vi "GPIB Bus Scan (for CCD).vi"(1 "Bus Timeout (mS)":i32=100) -> (0 "?":string)   [LabVIEW 2025]
doc: "Scans all primary addresses on the GPIB bus and reports status of devices found there.\nScott Hannahs, F. Bitter National Magnet Lab, April 1993\nAuthor: Scott Hannahs <sth@magnet.fsu.edu>\n\nThis software is licensed for use under the “MIT License\"\nCopyright (c) 2025 Scott Hannahs, sth@sth@magnet.sthnet.net\n\nPermission is hereby granted, free of charge, to any person obtaining a copy of this software and associated documentation files (the \"Software\"), to deal in the Software without restriction, including without limitation the rights to use, copy, modify, merge, publish, distribute, sublicense, and/or sell copies of the Software, and to permit persons to whom the Software is furnished to do so, subject to the following conditions: The above copyright notice and this permission notice shall be included in all copies or substantial portions of the Software.\n\nTHE SOFTWARE IS PROVIDED \"AS IS\", WITHOUT WARRANTY OF ANY KIND, EXPRESS OR IMPLIED, INCLUDING BUT NOT LIMITED TO THE WARRANTIES OF MERCHANTABILITY, FITNESS FOR A PARTICULAR PURPOSE AND NONINFRINGEMENT. IN NO EVENT SHALL THE AUTHORS OR COPYRIGHT HOLDERS BE LIABLE FOR ANY CLAIM, DAMAGES OR OTHER LIABILITY, WHETHER IN AN ACTION OF CONTRACT, TORT OR OTHERWISE, ARISING FROM, OUT OF OR IN CONNECTION WITH THE SOFTWARE OR THE USE OR OTHER DEALINGS IN THE SOFTWARE."
panel:
  in  "stop":bool
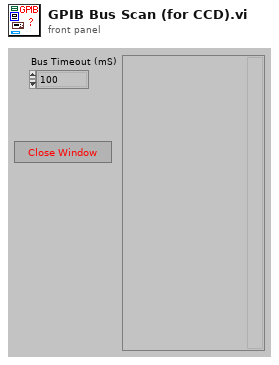
[diagram p1: front panel]
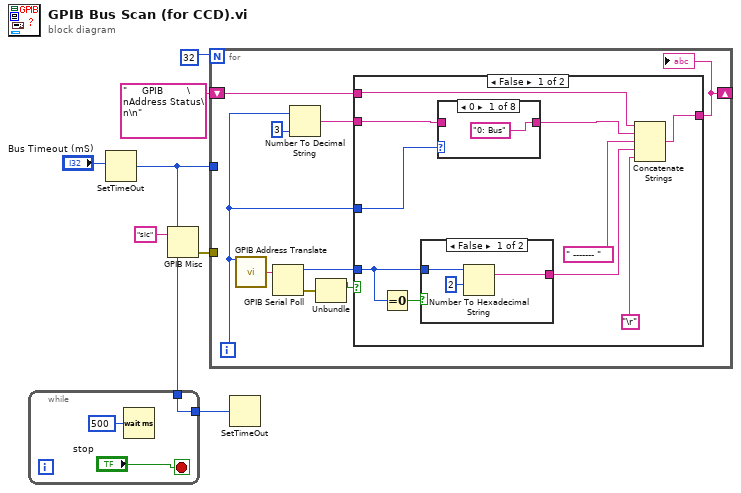
[diagram p0: block diagram]
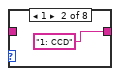
[diagram p2: hidden frame]
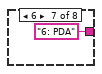
[diagram p7: hidden frame]
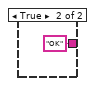
[diagram p9: hidden frame]
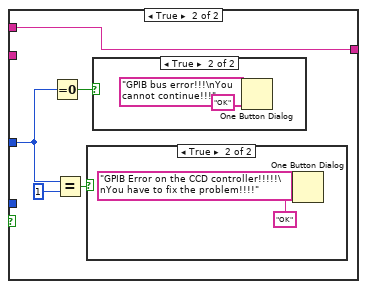
[diagram p10: hidden frame]
diagram:
  n1 = SetTimeOut(1:"Bus Timeout (mS)") -> (0:w2:i32)
  n2 = while {
    tunnel: [w8] -> w1
    tunnel: w2 -> [w8]
    stop <- "stop" stop-if-true
    n3 = Wait (ms)(milliseconds to wait=u32 500) -> ()  [unwired: 1 out]
  }
  n4 = GPIB Misc(0:"sic") -> (4:w4:errorcluster)  [unwired: 1 in, 2 out]
  n5 = for {
    N: 32 -> [_]
    shift-right: [w17] -> _
    shift-left: "     GPIB        \nAddress Status\n\n" -> [w19]
    tunnel: w2 -> [_]
    tunnel: w4 -> [_]
    i -> [w11]
    n6 = call "GPIB Address Translate.vi"("GPIB Address"=w11) -> ("GPIB Address String"=w16:string)
    n7 = GPIB Serial Poll(0:w16) -> (2:w18:i16, 4:w12:errorcluster)  [unwired: 1 in, 1 out]
    n8 = Number To Decimal String(number=w11, width (-)=3) -> (decimal integer string=w14:string)
    n9 = Unbundle(w12) -> ("status"=w13:bool)  [unwired: 2 out]
    n10 = case shown="False" w13 {
      tunnel: w18 -> [w24 _]
      tunnel: w14 -> [w21 _]
      tunnel: [w28 w46] -> w17
      tunnel: w19 -> [w29 w46]
      tunnel: w11 -> [w22 w43]
      frame False {
        n11 = Equal To 0?(x=w24) -> (x = 0?=w23:bool)
        n12 = case shown="False" w23 {
          tunnel: w24 -> [w40 _]
          tunnel: [w38 "OK"] -> w25
          frame False {
            n13 = Number To Hexadecimal String(1:2, 2:w40) -> (0:w38:string)
          }
          frame True {
          }
        }
        n14 = case shown="0" w22 {
          tunnel: w21 -> [_ _ w32 w33 w34 w35 _ w37]
          tunnel: ["0: Bus" "1: CCD" w32 w33 w34 w35 "6: PDA" w37] -> w20
          frame 0 {
          }
          frame 1 {
          }
          frame 2 {
          }
          frame 3 {
          }
          frame 4 {
          }
          frame 5 {
          }
          frame 6 {
          }
          frame 7, Default {
          }
        }
        n15 = Concatenate Strings(w29, w20, " ------- ", w25, "\r") -> (w28:string)
      }
      frame True {
        n16 = Equal To 0?(x=w43) -> (x = 0?=w45:bool)
        n17 = Equal?(x=w43, y=1) -> (x = y?=w44:bool)
        n18 = case shown="True" w44 {
          frame False {
          }
          frame True {
            n19 = One Button Dialog(message="GPIB Error on the CCD controller!!!!!\nYou have to fix the problem!!!!", button name ("OK")="OK") -> ()  [unwired: 1 out]
          }
        }
        n20 = case shown="True" w45 {
          frame False {
          }
          frame True {
            n21 = One Button Dialog(message="GPIB bus error!!!\nYou cannot continue!!!", button name ("OK")="OK") -> ()  [unwired: 1 out]
          }
        }
      }
    }
    "?" <- w17
  }
  n22 = SetTimeOut(1:w1) -> ()  [unwired: 1 out]
